vi "Read.vi"(8 "error in (no error)":errorcluster, 11 "Behavior in":refnum<class "BehaviorData.lvclass">) -> (0 "error out":errorcluster, 3 "Behavior out":refnum<class "BehaviorData.lvclass">)   [LabVIEW 2014, in "BehaviorData.lvclass"]
uses:
  BehaviorData.lvclass
  BehaviorData.lvclass/BehaviorData.ctl
panel:
  out "Backlog":u32
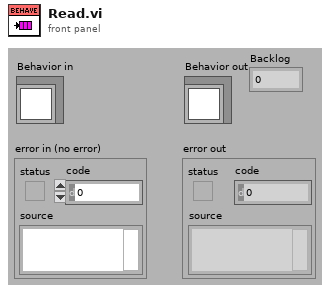
[diagram p1: front panel]
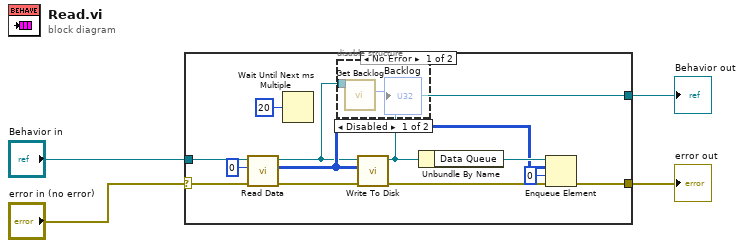
[diagram p0: block diagram]
diagram:
  n1 = case shown="No Error" "error in (no error)" {
    selector: "error in (no error)" -> [w15 w20]
    tunnel: [w9 w20] -> w3
    tunnel: [w6 w19] -> w1
    tunnel: "Behavior in" -> [w14 w19]
    frame No Error {
      n2 = call-dynamic "Read Data.vi"("error in (no error)"=w15, "Read Size"=0, "AcquireTraces in"=w14) -> ("error out"=w13:errorcluster, "data"=w10:i32[][], "AcquireTraces out"=w8:refnum<class "BehaviorData.lvclass">)  [unwired: 6 in]
      n3 = Wait Until Next ms Multiple(millisecond multiple=u32 20 ("milliseconds to wait")) -> ()  [unwired: 1 out]
      n4 = disable-structure shown="Disabled" {
        disable-tunnel: w8 -> [w18 _]
        frame Disabled {
          n5 = call-dynamic "Get Backlog.vi"("AcquireTraces in"=w18) -> ("Backlog"=→"Backlog":u32)  [unwired: 8 in, 2 out]
        }
        frame Enabled {
        }
      }
      n6 = call-dynamic "Write To Disk.vi"("error in (no error)"=w13, "element"=w10, "AcquireTraces in"=w8) -> ("error out"=w11:errorcluster, "AcquireTraces out"=w6:refnum<class "BehaviorData.lvclass">)  [unwired: 7 in]
      n7 = Unbundle By Name(w6) -> ("Data Queue"=w12:refnum<queue>)
      n8 = Enqueue Element(queue=w12, element=w10, timeout in ms (-1)=0, error in (no error)=w11) -> (error out=w9:errorcluster)  [unwired: 2 out]
    }
    frame Error {
    }
  }
  "error out" <- w3
  "Behavior out" <- w1
